vi "App Version.vi"() -> (1 "App Version":string)   [LabVIEW 2020, in "Volatus.lvlib" / "Volatus Core.lvclass"]
uses:
  Volatus Core.lvclass
  Volatus Core.lvclass/Volatus Core.ctl
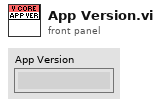
[diagram p1: front panel]
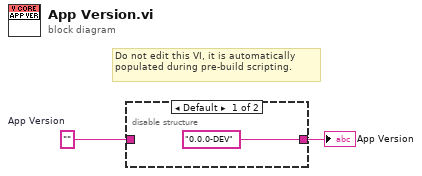
[diagram p0: block diagram]
diagram:
  w2 = ""  # App Version
  # "Do not edit this VI, it is automatically populated during pre-build scripting."
  n1 = disable-structure shown="Default" {
    disable-tunnel: w2 -> [_ w4]
    disable-tunnel: ["0.0.0-DEV" w4] -> w1
    frame condition #0 (active) {
    }
    frame condition #1 {
    }
  }
  "App Version" <- w1
